vi "Pivot Module.vi"(6 "Calibration Angle":dbl, 7 "Encoder Refnum":string="My AnalogChannel RefNum", 8 "Motor Speed":dbl, 9 "Motor Angle":dbl, 10 "Drive Motor Refnum":string="My Motor RefNum", 11 "Rotational Motor Refnum":string="My Motor RefNum") -> ()   [LabVIEW 2013]
uses:
  <vilib>/Rock Robotics/WPI/SafetyOutput/WPI_SafetyOutputConfigMenu.ctl
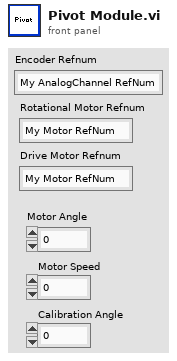
[diagram p1: front panel]
types:
  T1 = typedef "WPI_SafetyOutputConfigMenu.ctl" = enum16{"Enable", "Disable"}
  T2 = typedef "WPI_AnalogChannelDevRef.ctl" = cluster{"DevStatus":errorcluster, "Analog Module":T3, "Analog Channel":T4}
  T3 = typedef "FPGA_TypedefAnalogModule.ctl" = enum16{"Analog Module 1", "Analog Module 2"}
  T4 = typedef "FPGA_AIChannel.ctl" = enum8{"AI 1", "AI 2", "AI 3", "AI 4", "AI 5", "AI 6", "AI 7", "AI 8", "Invalid"}
  T5 = typedef "WPI_MotorControlDeviceRef.ctl" = cluster{"DeviceStatus":errorcluster, "Type":enum16{"PWM", "CAN"}, "PWM":cluster{"Digital Module":T6, "PWM Channel":T7, "DeadBand":T8}, "CAN":cluster{"Device Number":u8, "Control Mode":T9, "Semaphore":T10, "Max Vout":dbl}, "Invert":bool, "TransformRef":T11, "InvTransformRef":T11}
  T6 = typedef "FPGA_TypedefDigitalModule.ctl" = enum16{"Digital Module 1", "Digital Module 2"}
  T7 = typedef "FPGA_DIOPWMChannel.ctl" = enum8{"PWM 1", "PWM 2", "PWM 3", "PWM 4", "PWM 5", "PWM 6", "PWM 7", "PWM 8", "PWM 9", "PWM 10", "Invalid"}
  T8 = typedef "WPI_PWMDeadband.ctl" = cluster{"Name":string, "maxPositivePwm":i32, "minPositivePwm":i32, "centerPwm":i32, "maxNegativePwm":i32, "minNegativePwm":i32, "angularRange":u16}
  T9 = typedef "WPI_CANJaguar_ControlMode.ctl" = enum8{"Percent VBus", "Current", "Speed", "Position", "Voltage"}
  T10 = typedef "Semaphore RefNum" = refnum<k1>
  T11 = typedef "WPI_PWMTransform_ConPane.ctl" = refnum<vi>
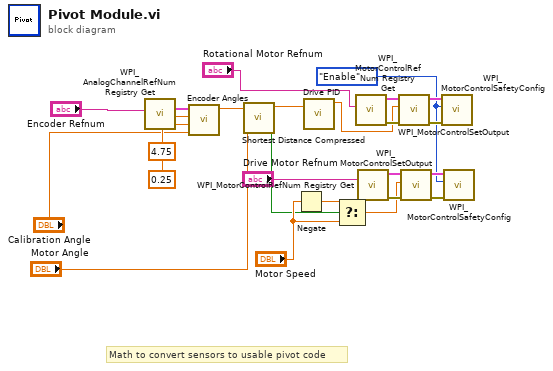
[diagram p0: block diagram]
diagram:
  w9 = WPI_SafetyOutputConfigMenu."Enable" ("mode")
  # "Math to convert sensors to usable pivot code"
  n1 = call <vilib>:"WPI_AnalogChannelRefNum Registry Get.vi"("refnum name"="Encoder Refnum") -> ("AIDeviceRef"=w8:T2)  [unwired: 9 in, 1 out]
  n2 = call "Encoder Angles.vi"("Calibration Angle"="Calibration Angle", "Bottom Voltage"=0.25, "Top Voltage"=4.75, "AIDeviceRef Encoder"=w8) -> ("Encoder Angle"=w4:dbl)  [unwired: 7 in]
  n3 = call "Shortest Distance Compressed.vi"("Needed angle"="Motor Angle", "Current Angle"=w4) -> ("Flip Motors?"=w1:bool, "Degrees to travel"=w2:dbl)  [unwired: 8 in]
  n4 = Negate(x="Motor Speed") -> (-x=w14:dbl)
  n5 = call "Drive PID.vi"("Process Variable"=w2) -> ("Output"=w19:dbl)  [unwired: 10 in]
  n6 = Select(t=w14, s=w1, f="Motor Speed") -> (s? t:f=w13:dbl)
  n7 = call <vilib>:"WPI_MotorControlRefNum Registry Get.vi"("refnum name"="Rotational Motor Refnum") -> ("error out"=w23:errorcluster, "MotorControlDevRef"=w22:T5)  [unwired: 9 in]
  n8 = call <vilib>:"WPI_MotorControlRefNum Registry Get.vi"("refnum name"="Drive Motor Refnum") -> ("error out"=w15:errorcluster, "MotorControlDevRef"=w16:T5)  [unwired: 9 in]
  n9 = call <vilib>:"WPI_MotorControlSetOutput.vi"("error in (no error)"=w23, "Output"=w19, "MotorControlDevRef"=w22) -> ("error out"=w20:errorcluster, "MotorControlDevRef"=w21:T5)  [unwired: 6 in, 1 out]
  n10 = call <vilib>:"WPI_MotorControlSetOutput.vi"("error in (no error)"=w15, "Output"=w13, "MotorControlDevRef"=w16) -> ("error out"=w18:errorcluster, "MotorControlDevRef"=w17:T5)  [unwired: 6 in, 1 out]
  n11 = call <vilib>:"WPI_MotorControlSafetyConfig.vi"("error in (no error)"=w20, "mode"=w9, "MotorControlDevRef"=w21) -> ()  [unwired: 7 in, 2 out]
  n12 = call <vilib>:"WPI_MotorControlSafetyConfig.vi"("error in (no error)"=w18, "mode"=w9, "MotorControlDevRef"=w17) -> ()  [unwired: 7 in, 2 out]
